vi "Moving_Average_of_5.vi"() -> ()   [LabVIEW 2019]
panel:
  out "Moving Average":dbl
  out "Current Number":dbl
  in  "stop":bool
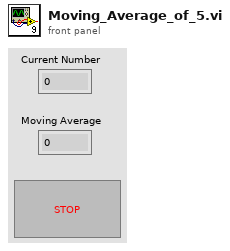
[diagram p1: front panel]
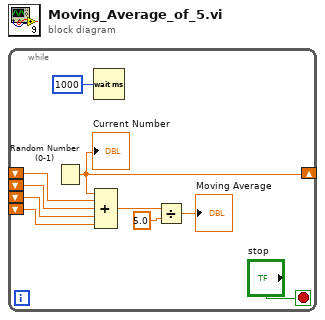
[diagram p0: block diagram]
diagram:
  n1 = while {
    shift-right: [w1] -> _
    shift-left: _ -> [w6]
    shift-left: _ -> [w5]
    shift-left: _ -> [w4]
    shift-left: _ -> [w3]
    stop <- "stop" stop-if-true
    n2 = Random Number (0-1)() -> (number: 0 to 1=w1:dbl)
    "Current Number" <- w1
    n3 = Wait (ms)(milliseconds to wait=u32 1000) -> ()  [unwired: 1 out]
    n4 = Compound Arithmetic op=ADD(w1, w6, w5, w4, w3) -> (w7:dbl)
    n5 = Divide(x=w7, y=5.0) -> (x/y=→"Moving Average":dbl)
  }
